vi "LDA_Analysis.vi"() -> (5 "Plug in titles":string[](array[string]), 7 "Plug in values":string[](array[string]))   [LabVIEW 2011]
uses:
  Controls/Save_Data.ctl
  Globals/LDA_meas_global_1.vi
  Globals/Plug_in_data_global.vi
  Globals/Meas_global.vi
  Globals/Constants_global.vi
  <vilib>/Analysis/NI_AALBase.lvlib
panel:
  in  "File Extension":string=".xls"
  out "Delta f":dbl
  in  "Refined Spectra":bool
  in  "No of estimates output":i32=300
  out "Autocorrelation":cluster{dbl, dbl, dbl[]}[](graph)
  in  "Mode":enum16{"Spectra", "Autocorrelation"}(ring)
  in  "Separation Character":string="\t"
  in  "Precision":i16=2
  out "Ch names":string[](array[string])
  out "Number or Good blocks":i32
  out "Resampled block length":i32
  out "Resampling Frequency":dbl
  in  "Output Directory":path
  in  "File":T1=enum."Save Data"
  out "Frequency Spectrum":cluster{dbl, dbl, dbl[]}[](graph)
  # "You must have just these two indicators on the connector pane of the vi"
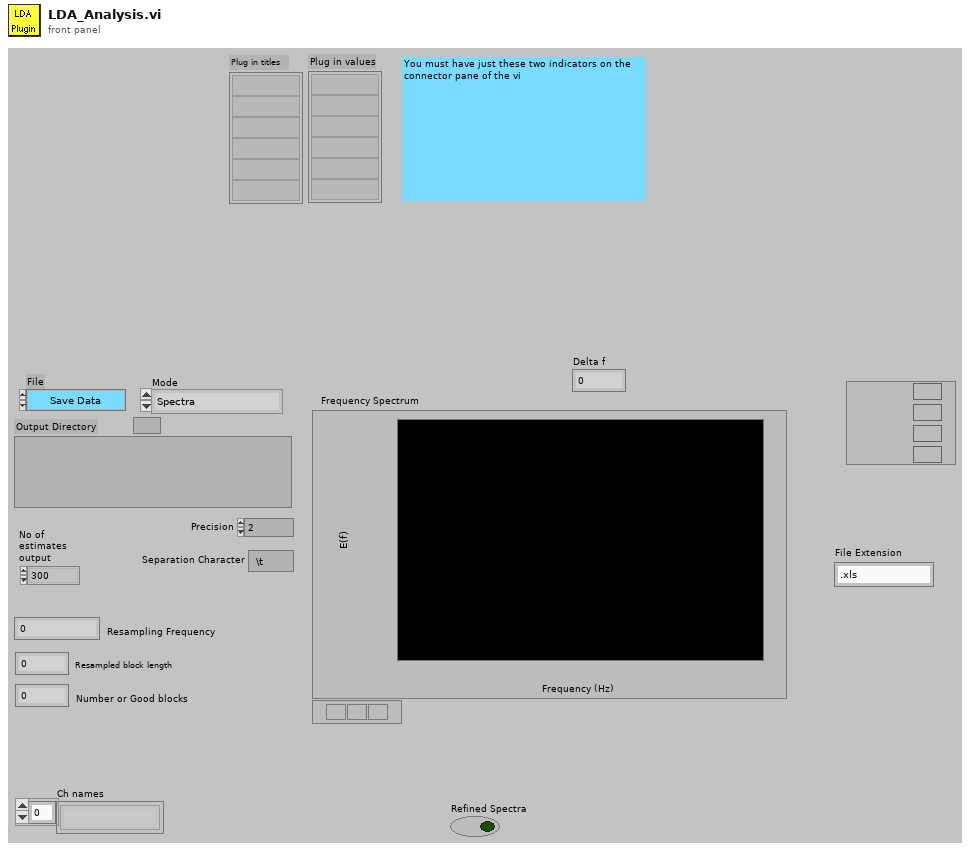
[diagram p1: front panel]
types:
  T1 = typedef "Save_Data.ctl" = enum16{"Save No Data", "Save Data"}
  T2 = enum32{"existing file", "new file", "new or existing file", "existing dir", "new dir", "new or existing dir", "existing file (use LLBs)", "new file (use LLBs)", "new or existing file (use LLBs)", "new or existing file or directory (use LLBs)"}
  T3 = typedef "Analysis_info_cluster.ctl" = cluster{"Colour":u32, "Inst type":T4, "Inst name":string, "Symbol":string, "Code name":string, "Extra Info":string, "Inst Array":T5, "Index":i32, "Voltage Index":i32, "Extra Titles":string[], "Extra Values":string[]}
  T4 = typedef "Inst_type.ctl" = enum16{"Propeller anemometer", "Raw voltage", "Pressure Transducer", "Pitot-static tube", "Preston tube", "Hot wire", "Cross wire 1", "Cross wire 2", "Generic Linear", "Generic Polynomial", "Generic BackPoly", "Fast FID", "Thermocouple", "Cold wire", "Pulsed Wire", "LDA Vel", "LDA Tran time", "LDA Arr time"}
  T5 = typedef "Instrument_Array.ctl" = enum16{"PWA", "LDA", "Analogue"}
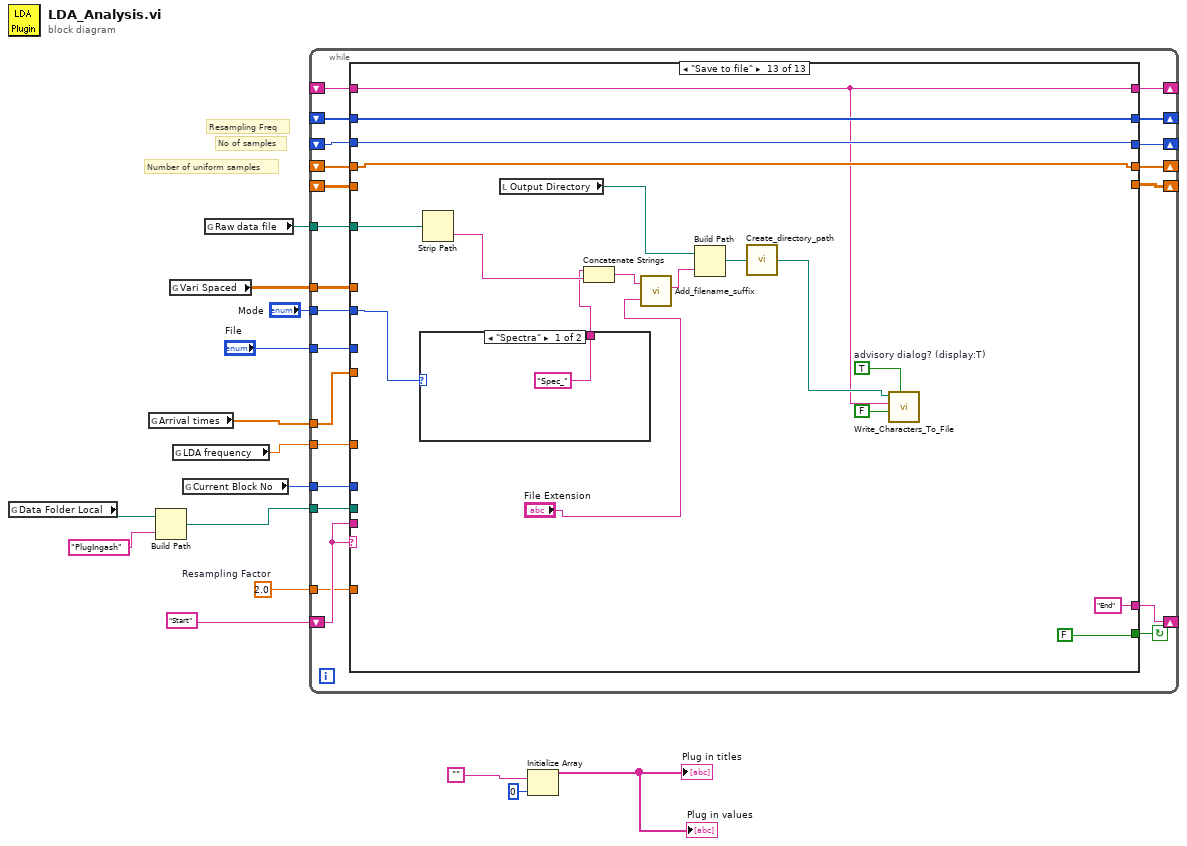
[diagram p0: block diagram]
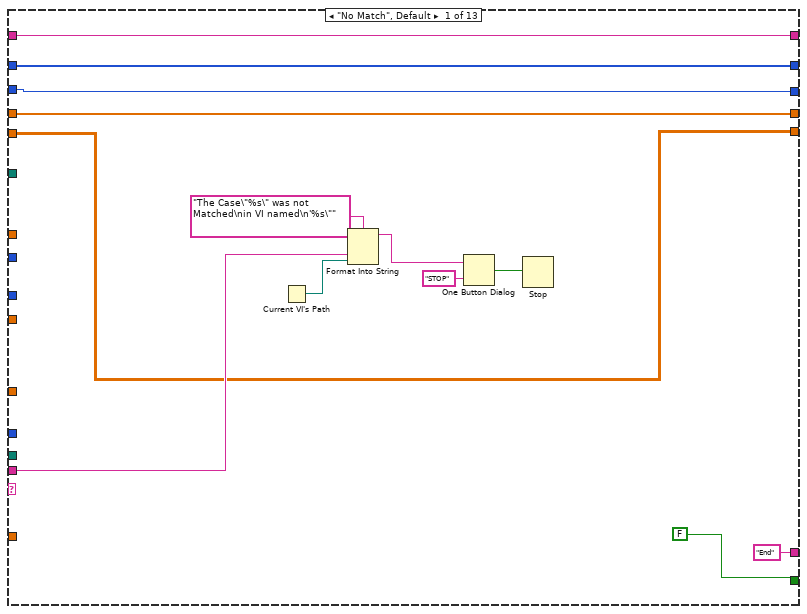
[diagram p2: hidden frame]
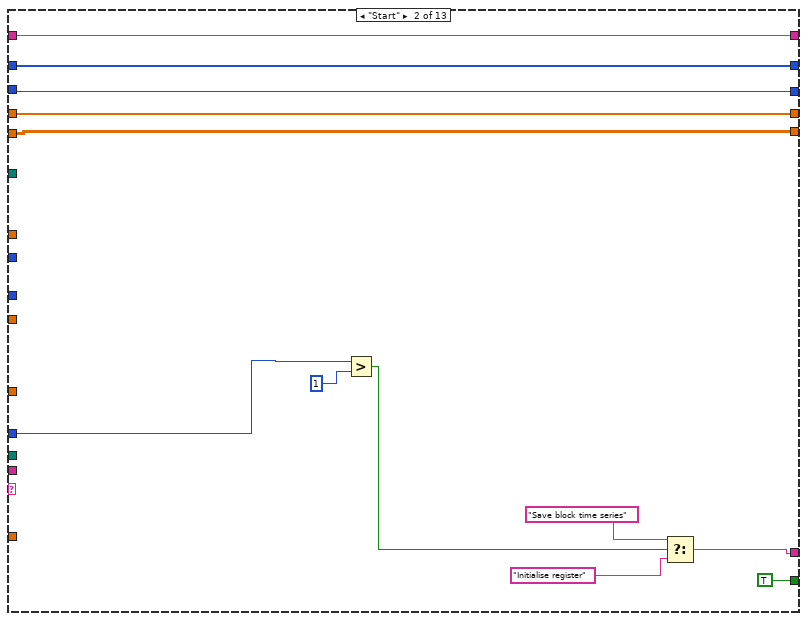
[diagram p3: hidden frame]
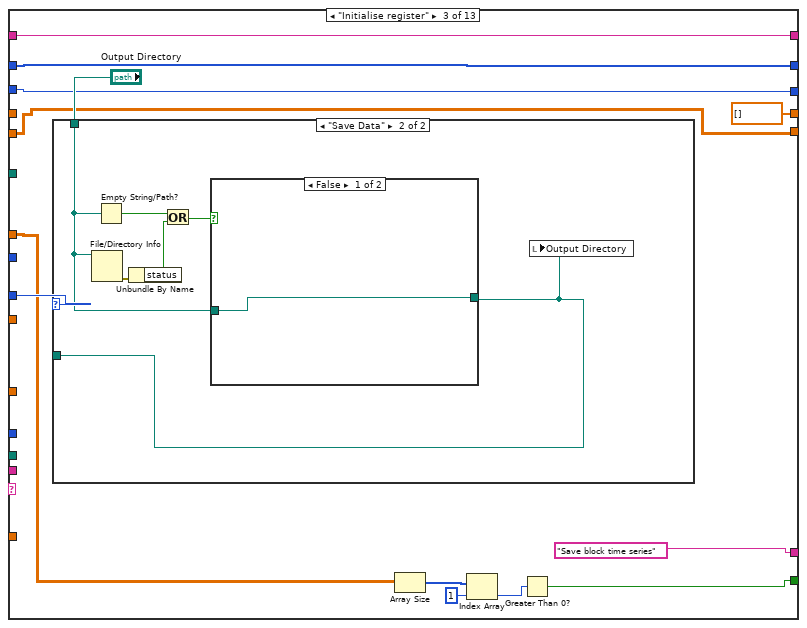
[diagram p4: hidden frame]
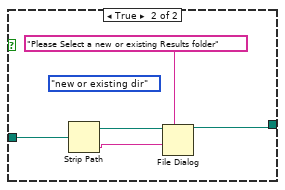
[diagram p6: hidden frame]
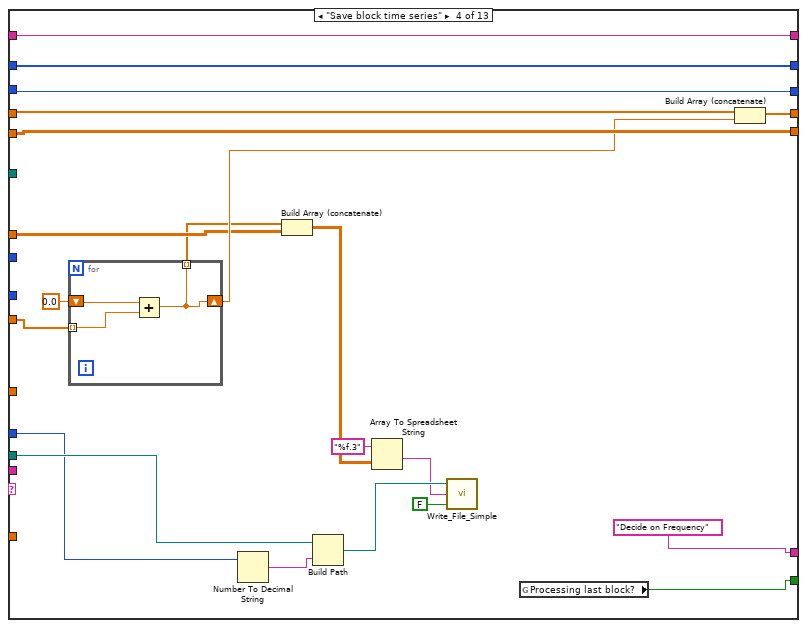
[diagram p7: hidden frame]
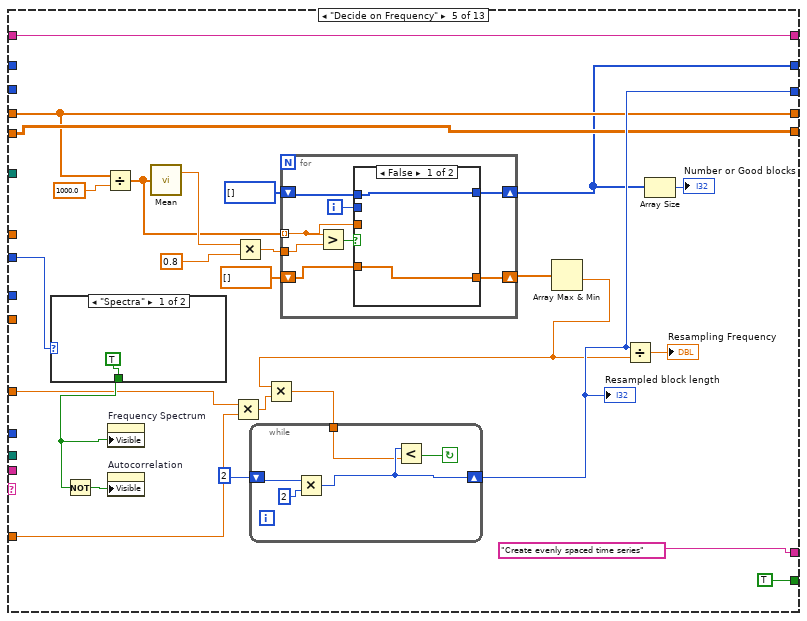
[diagram p8: hidden frame]
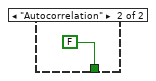
[diagram p9: hidden frame]
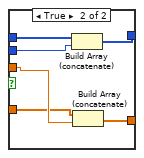
[diagram p10: hidden frame]
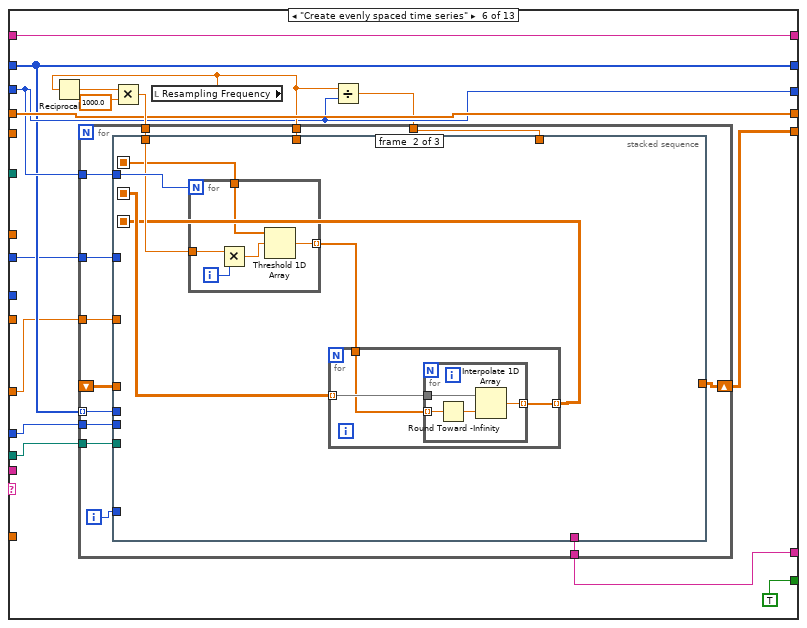
[diagram p11: hidden frame]
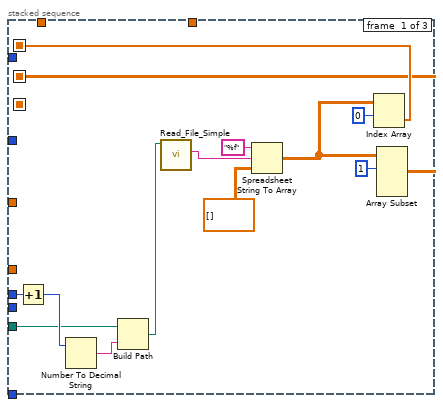
[diagram p12: hidden frame]
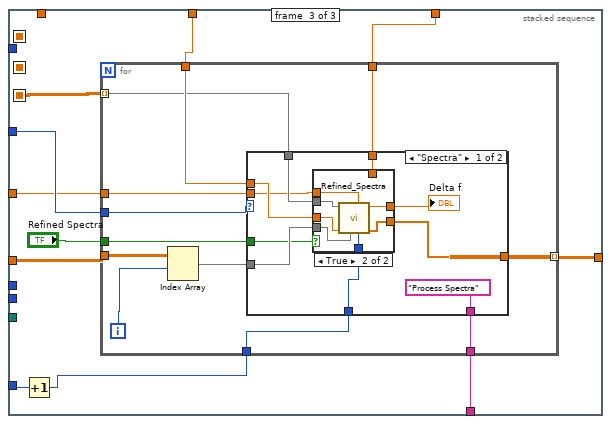
[diagram p13: hidden frame]
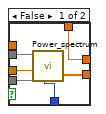
[diagram p14: hidden frame]
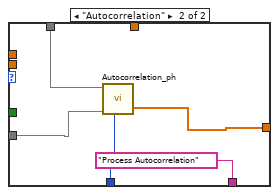
[diagram p15: hidden frame]
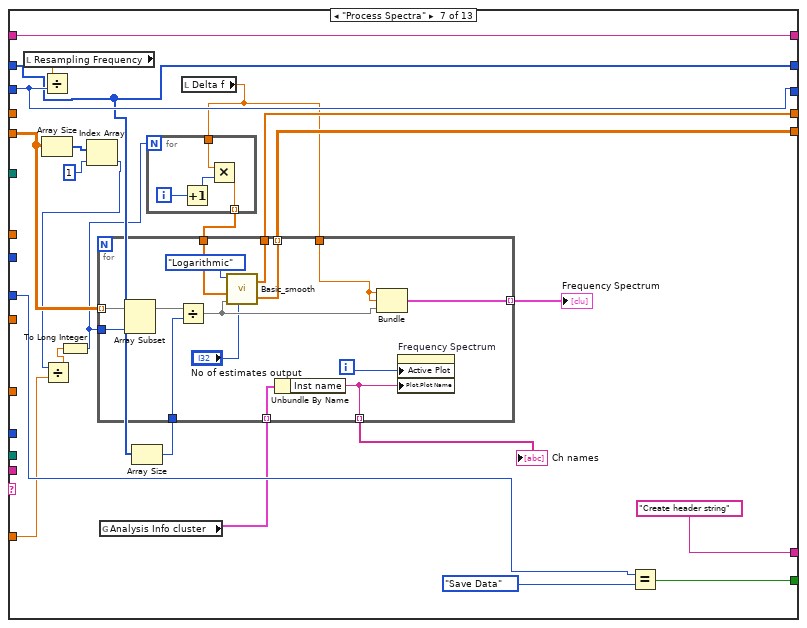
[diagram p16: hidden frame]
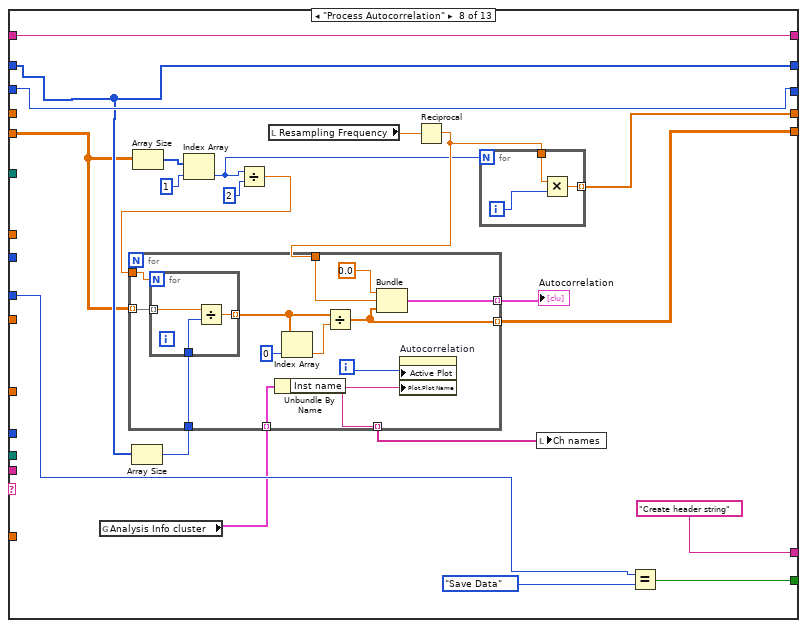
[diagram p17: hidden frame]
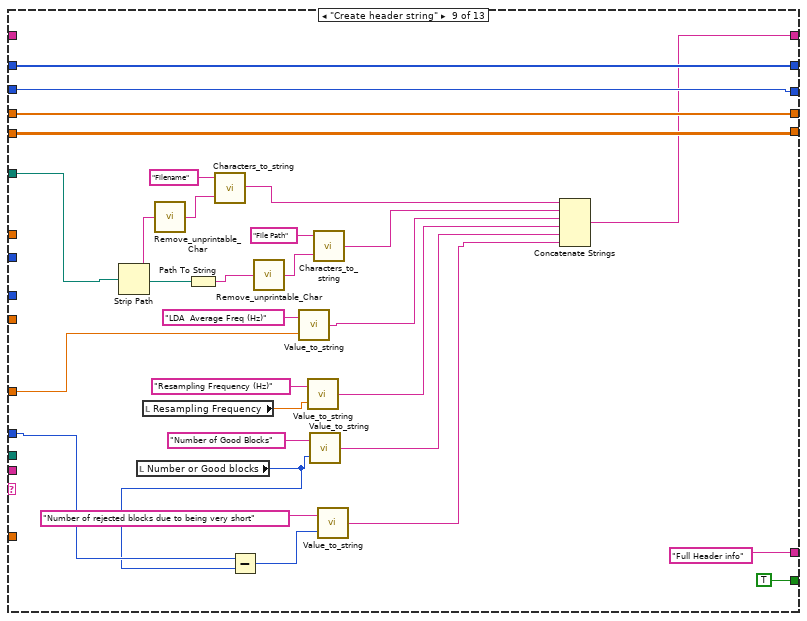
[diagram p18: hidden frame]
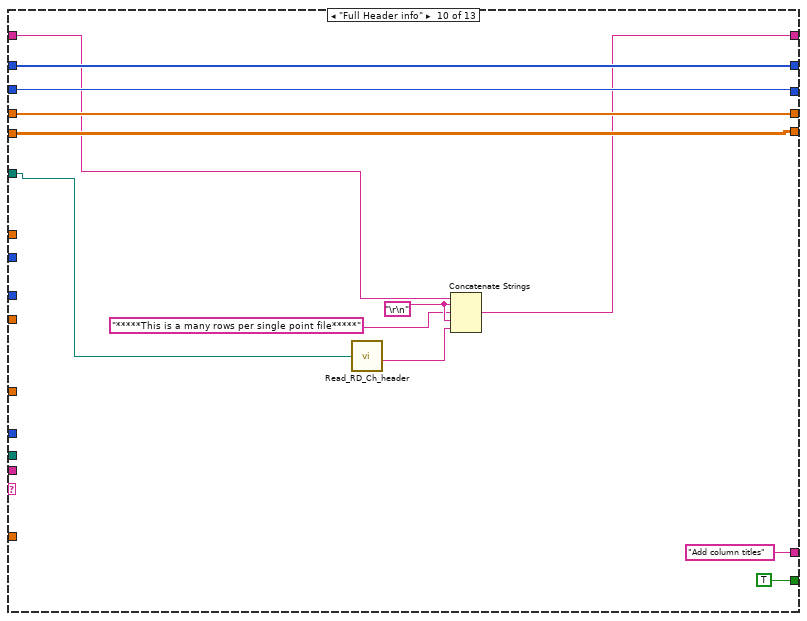
[diagram p19: hidden frame]
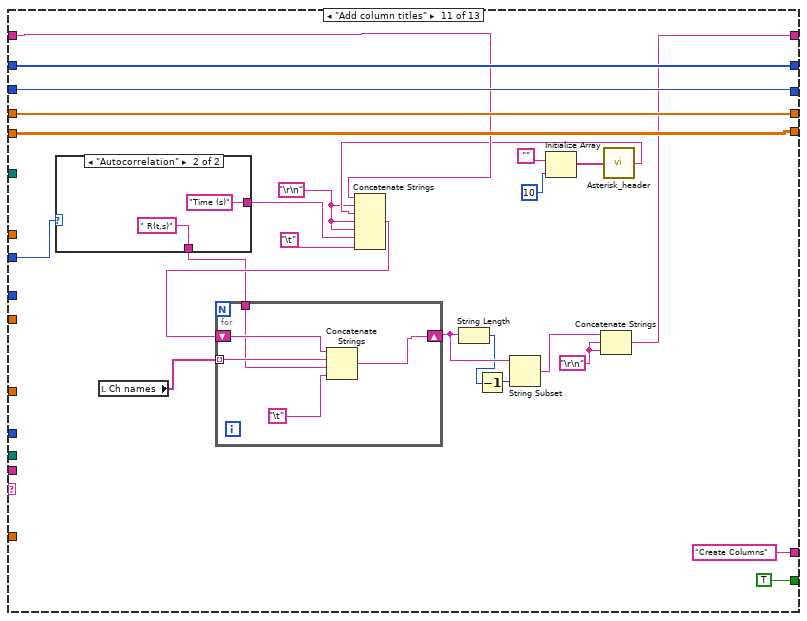
[diagram p20: hidden frame]
diagram:
  w1 = 2.0  # Resampling Factor
  # "No of samples"
  # "Number of uniform samples"
  # "Resampling Freq"
  n1 = global read "Constants_global.vi" "Data Folder Local"() -> (w7:path)
  n2 = global read "LDA_meas_global_1.vi" "Arrival times"() -> (w13:dbl[])
  n3 = Build Path(base path=w7, name or relative path="PlugIngash") -> (appended path=w6:path)
  n4 = global read "Plug_in_data_global.vi" "Vari Spaced"() -> (w14:dbl[][])
  n5 = global read "Meas_global.vi" "LDA frequency"() -> (w3:dbl)
  n6 = global read "Meas_global.vi" "Current Block No"() -> (w9:i32)
  n7 = global read "Meas_global.vi" "Raw data file"() -> (w4:path)
  n8 = while {
    shift-left: "Start" -> [w37]
    shift-right: [w34] -> _
    tunnel: w14 -> [w36]
    tunnel: w13 -> [w35]
    shift-right: [w32] -> _
    shift-left: _ -> [w31]
    shift-right: [w30] -> _
    shift-left: _ -> [w29]
    tunnel: w9 -> [w28]
    tunnel: w6 -> [w27]
    shift-right: [w26] -> _
    shift-left: _ -> [w25]
    tunnel: "File" -> [w24]
    shift-right: [w23] -> _
    shift-left: _ -> [w22]
    tunnel: w4 -> [w21]
    tunnel: w3 -> [w20]
    shift-right: [w19] -> _
    shift-left: _ -> [w18]
    tunnel: "Mode" -> [w17]
    tunnel: w1 -> [w16]
    stop <- w33 continue-if-true
    n9 = case shown="\"Save to file\"" w37 {
      tunnel: ["End" ("t") w57 "Save block time series" ("t") "Decide on Frequency" ("t") "Create evenly spaced time series" ("t") w164 "Create header string" "Create header string" "Full Header info" ("t") "Add column titles" ("t") "Create Columns" ("t") "Save to file" ("t") "End" ("t")] -> w34
      tunnel: w37 -> [w46 _ _ _ _ _ _ _ _ _ _ _ _]
      tunnel: w36 -> [_ _ w67 w90 _ _ _ _ _ _ _ _ _]
      tunnel: w35 -> [_ _ _ w96 _ _ _ _ _ _ _ _ _]
      tunnel: [FALSE TRUE w63 w101 TRUE TRUE ("Processing last block?") w290 w331 TRUE ("Processing last block?") TRUE ("Processing last block?") TRUE ("Processing last block?") TRUE ("Processing last block?") FALSE] -> w33
      tunnel: [w43 w53 w70 w97 w131 w173 w286 w325 w358 w393 w417 w435 _] -> w32
      tunnel: w31 -> [w43 w53 w70 w97 w131 _ w279 w322 w358 w393 w417 w435 _]
      tunnel: [w41 w56 dbl[] [] w99 w127 w172 w282 w316 w359 w394 w418 w430 w491] -> w30
      tunnel: w29 -> [w41 w56 _ w100 w127 w172 _ _ w359 w394 w418 w430 w491]
      tunnel: w28 -> [_ w55 _ w106 _ w162 _ _ w367 _ _ _ _]
      tunnel: w27 -> [_ _ _ w107 _ w175 _ _ _ _ _ _ _]
      tunnel: [w42 w54 w71 w98 w132 w169 w293 w334 w360 w395 w419 w437 w492] -> w26
      tunnel: w25 -> [w42 w54 w71 w98 _ w169 w293 w334 w360 w395 w419 w437 w492]
      tunnel: w24 -> [_ _ w72 _ _ _ w291 w332 _ _ _ _ _]
      tunnel: [w40 w52 w69 w93 w121 w167 w285 w328 w361 w396 w420 w445 w490] -> w23
      tunnel: w22 -> [w40 w52 w69 w93 _ w167 w285 w328 w361 w396 w420 w445 w490]
      tunnel: w21 -> [_ _ _ _ _ _ _ _ w373 w386 _ _ w489]
      tunnel: w20 -> [_ _ _ _ w114 w163 _ _ w370 _ _ _ _]
      tunnel: [w39 w51 w68 w92 w119 w166 w289 w330 w357 w385 w413 w441 w482] -> w19
      tunnel: w18 -> [w39 w51 w68 w92 w119 w166 w289 w330 _ w392 w407 w442 w482]
      tunnel: w17 -> [_ _ _ _ w118 w165 _ _ _ _ w410 _ w479]
      tunnel: w16 -> [_ _ _ _ w113 _ w275 _ _ _ _ _ _]
      frame "No Match", Default {
        n10 = Current VI's Path() -> (path=w45:path)
        n11 = Format Into String(format string="The Case\"%s\" was not Matched\nin VI named\n'%s\"" ("Format String"), w46, w45) -> (resulting string=w49:string)  [unwired: 2 in, 1 out]
        n12 = One Button Dialog(message=w49, button name ("OK")="STOP") -> (true=w47:bool)
        n13 = Stop(stop? (T)=w47) -> ()
      }
      frame "Start" {
        n14 = Greater?(x=w55, y=1) -> (0:w59:bool)
        n15 = Select(t="Save block time series", s=w59, f="Initialise register") -> (s? t:f=w57:string)
      }
      frame "Initialise register" {
        n16 = case shown="\"Save Data\"" w72 {
          tunnel: [w76 w82] -> _
          tunnel: "Output Directory" -> [w76 w80]
          frame "Save No Data" {
          }
          frame "Save Data" {
            n17 = File/Directory Info(path=w80) -> (error out=w81:errorcluster)  [unwired: 1 in, 6 out]
            n18 = Empty String/Path?(string/path=w80) -> (empty?=w78:bool)
            n19 = Unbundle By Name(w81) -> ("status"=w79:bool)
            n20 = Or(x=w78, y=w79) -> (x .or. y?=w77:bool)
            n21 = case shown="False" w77 {
              tunnel: [w83 w88] -> w82
              tunnel: w80 -> [w83 w86]
              frame False {
              }
              frame True {
                (unwired) T2."new or existing dir" ("select mode (2)")
                n22 = Strip Path(path=w86) -> (stripped path=w85:path, name=w84:string)
                n23 = File Dialog(7:"Please Select a new or existing Results folder" ("prompt"), 9:w84, 11:w85) -> (3:w88:path)  [unwired: 1 in, 6 out]
              }
            }
            n24 = local write "Output Directory"(w82) -> ()
          }
        }
        n25 = Array Size(array=w67) -> (size(s)=w66:i32[])
        n26 = Index Array(array=w66, index=1) -> (element=w64:i32)
        n27 = Greater Than 0?(x=w64) -> (x > 0?=w63:bool)
      }
      frame "Save block time series" {
        n28 = for {
          shift-right: [w110] -> w94
          shift-left: 0.0 -> [w112]
          tunnel: w96 -> [w111] mode=indexing
          tunnel: [w110] -> w89 mode=indexing
          n29 = Add(x=w112, y=w111) -> (x+y=w110:dbl)
        }
        n30 = Number To Decimal String(number=w106) -> (decimal integer string=w105:string)  [unwired: 1 out]
        n31 = Build Array (concatenate)(w89, w90) -> (w91:dbl[][])
        n32 = Build Path(base path=w107, name or relative path=w105) -> (appended path=w104:path)
        n33 = Array To Spreadsheet String(array=w91, 3:"%f.3" ("format string")) -> (spreadsheet string=w103:string)  [unwired: 1 out]
        n34 = call "Write_File_Simple.vi"("append to file? (new file:F)"=FALSE, "character string"=w103, "file path"=w104) -> ()  [unwired: 2 out]
        n35 = global read "Meas_global.vi" "Processing last block?"() -> (w101:bool)
        n36 = Build Array (concatenate)(w100, w94) -> (w99:dbl[])
      }
      frame "Decide on Frequency" {
        n37 = case shown="\"Spectra\"" w118 {
          tunnel: [TRUE FALSE] -> w116
          frame "Spectra" {
          }
          frame "Autocorrelation" {
          }
        }
        n38 = Not(x=w116) -> (.not. x?=w117:bool)
        n39 = Divide(x=w127, y=1000.0) -> (x/y=w125:dbl[])
        n40 = property on="Frequency Spectrum" class="WFGraph (strict)"("Visible"=w116) -> ()  [unwired: 2 in, 2 out]
        n41 = property on="Autocorrelation" class="WFGraph (strict)"("Visible"=w117) -> ()  [unwired: 2 in, 2 out]
        n42 = call <vilib>:"Mean.vi"("X"=w125) -> ("mean"=w130:dbl)  [unwired: 1 out]
        n43 = Multiply(x=w114, y=w113) -> (x*y=w115:dbl)
        n44 = Multiply(x=w130, y=0.8) -> (x*y=w128:dbl)
        n45 = for {
          tunnel: w125 -> [w143] mode=indexing
          tunnel: w128 -> [w148]
          shift-right: [w144] -> w121
          shift-left: i32[] [] -> [w145]
          shift-right: [w141] -> w123
          shift-left: dbl[] [] -> [w142]
          i -> [w146]
          n46 = Greater?(x=w143, y=w148) -> (0:w147:bool)
          n47 = case shown="False" w147 {
            tunnel: w146 -> [_ w156]
            tunnel: w145 -> [w150 w155]
            tunnel: [w150 w154] -> w144
            tunnel: w143 -> [_ w153]
            tunnel: w142 -> [w149 w152]
            tunnel: [w149 w151] -> w141
            frame False {
            }
            frame True {
              n48 = Build Array (concatenate)(w155, w156) -> (w154:i32[])
              n49 = Build Array (concatenate)(w152, w153) -> (w151:dbl[])
            }
          }
        }
        n50 = Array Max & Min(array=w123) -> (min value=w122:dbl)  [unwired: 3 out]
        n51 = Multiply(x=w122, y=w115) -> (x*y=w134:dbl)
        n52 = while {
          shift-right: [w159] -> w132
          shift-left: 2 -> [w161]
          tunnel: w134 -> [w158]
          stop <- w157 continue-if-true
          n53 = Multiply(x=w161, y=2) -> (x*y=w159:i32)
          n54 = Less?(x=w159, y=w158) -> (x < y?=w157:bool)
        }
        "Resampled block length" <- w132
        n55 = Divide(x=w132, y=w122) -> (x/y=→"Resampling Frequency":dbl)
        n56 = Array Size(array=w121) -> (size(s)=→"Number or Good blocks":i32)
      }
      frame "Create evenly spaced time series" {
        n57 = local read "Resampling Frequency"() -> (w170:dbl)
        n58 = Reciprocal(x=w170) -> (1/x=w176:dbl)
        n59 = Multiply(x=w176, y=1000.0) -> (x*y=w174:dbl)
        n60 = Divide(x=w170, y=w169) -> (x/y=w168:dbl)
        n61 = for {
          tunnel: w175 -> [w190]
          tunnel: w169 -> [w189]
          tunnel: w174 -> [w188]
          shift-right: [w186] -> w173
          shift-left: _ -> [w187]
          tunnel: w170 -> [w185]
          tunnel: w168 -> [w184]
          tunnel: w167 -> [w182] mode=indexing
          tunnel: w165 -> [w181]
          tunnel: [w180] -> w164
          tunnel: w163 -> [w179]
          tunnel: w162 -> [w178]
          i -> [w183]
          n62 = stacked-sequence {
            seq-local: [w196 _ _] -> [_ w207 _]
            seq-local: [w193 _ _] -> [_ w205 _]
            seq-local: [_ w204 _] -> [_ _ w232]
            tunnel: w183 -> [_ _ w228]
            tunnel: w190 -> [w201 _ _]
            tunnel: w189 -> [_ w209 _]
            tunnel: w188 -> [_ w208 _]
            tunnel: w187 -> [_ _ w231]
            tunnel: [_ _ w230] -> w186
            tunnel: w185 -> [_ _ w229]
            tunnel: w184 -> [_ _ w222]
            tunnel: w182 -> [w191 _ _]
            tunnel: w181 -> [_ _ w226]
            tunnel: [_ _ w225] -> w180
            tunnel: w179 -> [_ _ w224]
            tunnel: w178 -> [_ _ _]
            frame #0 {
              n63 = Increment(x=w191) -> (x+1=w202:i32)
              n64 = Number To Decimal String(number=w202) -> (decimal integer string=w203:string)  [unwired: 1 out]
              n65 = Build Path(base path=w201, name or relative path=w203) -> (appended path=w200:path)
              n66 = call "Read_File_Simple.vi"("Filename"=w200) -> ("string"=w199:string)  [unwired: 2 in, 7 out]
              n67 = Spreadsheet String To Array(format string="%f", spreadsheet string=w199, array type (2D Dbl)=dbl[][] []) -> (array=w195:dbl[][])  [unwired: 1 out]
              n68 = Index Array(array=w195, index (row)=0) -> (element=w196:dbl[])  [unwired: 1 in]
              n69 = Array Subset(array=w195, index (row)=1 ("index")) -> (w193:dbl[][])  [unwired: 3 in]
            }
            frame #1 {
              n70 = for {
                N: w209 -> [_]
                tunnel: w208 -> [w220]
                tunnel: w207 -> [w219]
                tunnel: [w218] -> w206 mode=indexing
                i -> [w221]
                n71 = Multiply(x=w220, y=w221) -> (x*y=w217:dbl)
                n72 = Threshold 1D Array(2:w217, 3:w219) -> (0:w218:dbl)  [unwired: 1 out]
              }
              n73 = for {
                tunnel: [w212] -> w204 mode=indexing
                tunnel: w206 -> [w210]
                tunnel: w205 -> [w211] mode=indexing
                n74 = for {
                  tunnel: w211 -> [w216]
                  tunnel: w210 -> [w215] mode=indexing
                  tunnel: [w214] -> w212 mode=indexing
                  n75 = Round Toward -Infinity(1:w215) -> (0:w213:dbl)
                  n76 = Interpolate 1D Array(1:w213, 2:w216) -> (0:w214:dbl)
                }
              }
            }
            frame #2 {
              n77 = Increment(x=w228) -> (x+1=w227:i32)
              n78 = for {
                tunnel: w232 -> [w240] mode=indexing
                tunnel: [w239] -> w230 mode=indexing
                tunnel: w231 -> [w244]
                tunnel: w229 -> [w241]
                tunnel: w227 -> [w238]
                tunnel: w226 -> [w237]
                tunnel: [w236] -> w225
                tunnel: w224 -> [w235]
                tunnel: "Refined Spectra" -> [w234]
                tunnel: w222 -> [w233]
                i -> [w242]
                n79 = Index Array(array=w244, index (row)=w242) -> (element=w243:dbl[])  [unwired: 1 in]
                n80 = case shown="\"Spectra\"" w237 {
                  tunnel: w243 -> [w254 w271]
                  tunnel: w241 -> [w249 _]
                  tunnel: w240 -> [w250 w272]
                  tunnel: [w253 w270] -> w239
                  tunnel: w238 -> [w252 w269]
                  tunnel: ["Process Spectra" ("t") "Process Autocorrelation" ("t")] -> w236
                  tunnel: w235 -> [w248 _]
                  tunnel: w234 -> [w247 _]
                  tunnel: w233 -> [w245 _]
                  frame "Spectra" {
                    n81 = case shown="True" w247 {
                      tunnel: w254 -> [w260 w264]
                      tunnel: [w259 w266] -> w253
                      tunnel: w252 -> [w258 w263]
                      tunnel: w250 -> [w257 w267]
                      tunnel: w249 -> [w256 w265]
                      tunnel: w248 -> [_ w262]
                      tunnel: [w255 w261] -> w246
                      tunnel: w245 -> [w255 _]
                      frame False {
                        n82 = call "Power_spectrum.vi"("U"=w257, "Sampling frequency"=w256, "Spectrum input array"=w260, "Block No"=w258) -> ("Spectrum output array"=w259:dbl[])  [unwired: 1 in, 1 out]
                      }
                      frame True {
                        n83 = call "Refined_Spectra.vi"("Block No"=w263, "LDA Frequency"=w262, "Spectrum input array"=w264, "Sampling frequency"=w265, "X"=w267) -> ("Spectrum"=w266:dbl[], "Delta f"=w261:dbl)  [unwired: 5 in]
                      }
                    }
                    "Delta f" <- w246
                  }
                  frame "Autocorrelation" {
                    n84 = call "Autocorrelation_ph.vi"("X"=w272, "Autocorrelation of X"=w271, "Block No"=w269) -> ("Autocorrelation of X"=w270:dbl[])  [unwired: 2 in, 1 out]
                  }
                }
              }
            }
          }
        }
      }
      frame "Process Spectra" {
        (unwired) FALSE
        n85 = local read "Resampling Frequency"() -> (w294:dbl)
        n86 = Divide(x=w294, y=w293) -> ()  [unwired: 1 out]
        n87 = Array Size(array=w279) -> (size(s)=w281:i32[])
        n88 = Index Array(array=w281, index=1) -> (element=w276:i32)
        n89 = Divide(x=w276, y=w275) -> (x/y=w274:dbl)
        n90 = To Long Integer(number=w274) -> (32bit integer=w273:i32)
        n91 = global read "Meas_global.vi" "Analysis Info cluster"() -> (w287:T3[])
        n92 = Array Size(array=w285) -> (size(s)=w284:i32)
        n93 = local read "Delta f"() -> (w278:dbl)
        n94 = for {
          N: w273 -> [_]
          tunnel: w278 -> [w297]
          tunnel: [w296] -> w283 mode=indexing
          i -> [w299]
          n95 = Increment(x=w299) -> (x+1=w298:i32)
          n96 = Multiply(x=w297, y=w298) -> (x*y=w296:dbl)
        }
        n97 = for {
          tunnel: w279 -> [w301] mode=indexing
          tunnel: w284 -> [w314]
          tunnel: [w313] -> w277 mode=indexing
          tunnel: w287 -> [w311] mode=indexing
          tunnel: [w310] -> w288 mode=indexing
          tunnel: [w305] -> w286 mode=indexing
          tunnel: w283 -> [w308]
          tunnel: [w304] -> w282
          tunnel: w278 -> [w303]
          tunnel: w273 -> [w300]
          i -> [w312]
          n98 = Array Subset(array=w301, length=w300) -> (w302:dbl[])  [unwired: 1 in]
          n99 = Divide(x=w302, y=w314) -> (x/y=w309:dbl[])
          n100 = call "Basic_smooth.vi"("Smoothing"=enum16{"Linear", "Logarithmic"}."Logarithmic", "X array in"=w308, "Y array in"=w309, "No of estimates output"="No of estimates output") -> ("X array Out"=w304:dbl[], "Y array Out"=w305:dbl[])  [unwired: 1 out]
          n101 = Unbundle By Name(w311) -> ("Inst name"=w310:string)
          n102 = Bundle("Delta f"=w303, "Delta f"=w303, w309) -> (w313:cluster{"Delta f":dbl, "Delta f":dbl, dbl[]})  [unwired: 1 out]
          n103 = property on="Frequency Spectrum" class="WFGraph (strict)"("Active Plot"=w312, "Plot.Plot Name"=w310) -> ()  [unwired: 2 in, 2 out]
        }
        "Frequency Spectrum" <- w277
        "Ch names" <- w288
        n104 = Equal?(x=w291, y=Save_Data."Save Data" ("File")) -> (x = y?=w290:bool)
      }
      frame "Process Autocorrelation" {
        (unwired) FALSE
        n105 = global read "Meas_global.vi" "Analysis Info cluster"() -> (w329:T3[])
        n106 = Array Size(array=w328) -> (size(s)=w327:i32)
        n107 = Array Size(array=w322) -> (size(s)=w321:i32[])
        n108 = Index Array(array=w321, index=1) -> (element=w315:i32)
        n109 = Divide(x=w315, y=2) -> (x/y=w318:dbl)
        n110 = local read "Resampling Frequency"() -> (w326:dbl)
        n111 = Reciprocal(x=w326) -> (1/x=w317:dbl)
        n112 = for {
          tunnel: w317 -> [w351]
          tunnel: w322 -> [w350] mode=indexing
          tunnel: w327 -> [w349]
          tunnel: [w348] -> w323 mode=indexing
          tunnel: w329 -> [w347] mode=indexing
          tunnel: [w342] -> w325 mode=indexing
          tunnel: [w340] -> w324 mode=indexing
          tunnel: w318 -> [w339]
          i -> [w341]
          n113 = for {
            N: w339 -> [_]
            tunnel: w350 -> [w354] mode=indexing
            tunnel: w349 -> [w353]
            tunnel: [w352] -> w344 mode=indexing
            n114 = Divide(x=w354, y=w353) -> (x/y=w352:dbl)
          }
          n115 = Unbundle By Name(w347) -> ("Inst name"=w340:string)
          n116 = Index Array(array=w344, index=0) -> (element=w343:dbl)
          n117 = Divide(x=w344, y=w343) -> (x/y=w342:dbl[])
          n118 = Bundle(0.0, w351, w342) -> (w348:cluster{dbl, dbl, dbl[]})  [unwired: 1 out]
          n119 = property on="Autocorrelation" class="WFGraph (strict)"("Active Plot"=w341, "Plot.Plot Name"=w340) -> ()  [unwired: 2 in, 2 out]
        }
        "Autocorrelation" <- w323
        n120 = for {
          N: w315 -> [_]
          tunnel: w317 -> [w338]
          tunnel: [w336] -> w316 mode=indexing
          i -> [w337]
          n121 = Multiply(x=w338, y=w337) -> (x*y=w336:dbl)
        }
        n122 = local write "Ch names"(w324) -> ()
        n123 = Equal?(x=w332, y=Save_Data."Save Data" ("File")) -> (x = y?=w331:bool)
      }
      frame "Create header string" {
        n124 = Strip Path(path=w373) -> (stripped path=w377:path, name=w381:string)
        n125 = local read "Number or Good blocks"() -> (w366:i32)
        n126 = local read "Resampling Frequency"() -> (w369:dbl)
        n127 = call "Remove_unprintable_Char.vi"("Input String"=w381) -> ("Output String"=w380:string)
        n128 = Path To String(path=w377) -> (string=w376:string)
        n129 = call "Characters_to_string.vi"("Characters to write"=w380, "Label for characters"="Filename") -> ("Output string"=w375:string)
        n130 = Subtract(x=w367, y=w366) -> (x-y=w365:i32)
        n131 = call "Remove_unprintable_Char.vi"("Input String"=w376) -> ("Output String"=w379:string)
        n132 = call "Value_to_string.vi"("Value"=w370, "Label for value"="LDA  Average Freq (Hz)") -> ("Output string"=w384:string)  [unwired: 1 in]
        n133 = call "Value_to_string.vi"("Value"=w369, "Label for value"="Resampling Frequency (Hz)") -> ("Output string"=w364:string)  [unwired: 1 in]
        n134 = call "Value_to_string.vi"("Value"=w366, "Label for value"="Number of Good Blocks") -> ("Output string"=w363:string)  [unwired: 1 in]
        n135 = call "Characters_to_string.vi"("Characters to write"=w379, "Label for characters"="File Path") -> ("Output string"=w374:string)
        n136 = call "Value_to_string.vi"("Value"=w365, "Label for value"="Number of rejected blocks due to being very short") -> ("Output string"=w362:string)  [unwired: 1 in]
        n137 = Concatenate Strings(w375, w374, w384, w364, w363, w362) -> (w357:string)
      }
      frame "Full Header info" {
        w389 = "\r\n"
        n138 = call "Read_RD_Ch_header.vi"("Raw data file"=w386) -> ("Ch string"=w387:string)  [unwired: 3 out]
        n139 = Concatenate Strings(w392, w389, "*****This is a many rows per single point file*****", w389, w387) -> (w385:string)
      }
      frame "Add column titles" {
        w401 = "\r\n"
        w402 = "\r\n"
        n140 = case shown="\"Autocorrelation\"" w410 {
          tunnel: ["f (Hz)" "Time (s)"] -> w409
          tunnel: [" E(f)" " R(t,s)"] -> w408
          frame "Spectra" {
          }
          frame "Autocorrelation" {
          }
        }
        n141 = local read "Ch names"() -> (w415:string[])
        n142 = Initialize Array("", 10) -> (w406:string[])
        n143 = call "Asterisk_header.vi"("Channel names"=w406) -> ("Header string"=w403:string)
        n144 = Concatenate Strings(w407, w401, w403, w401, w401, w409, "\t") -> (w414:string)
        n145 = for {
          shift-right: [w426] -> w400
          shift-left: w414 -> [w428]
          tunnel: w415 -> [w429] mode=indexing
          tunnel: w408 -> [w425]
          n146 = Concatenate Strings(w428, w429, w425, "\t") -> (w426:string)
        }
        n147 = String Length(string=w400) -> (length=w397:i32)
        n148 = Decrement(x=w397) -> (x-1=w398:i32)
        n149 = String Subset(string=w400, length (rest)=w398) -> (substring=w399:string)  [unwired: 1 out]
        n150 = Concatenate Strings(w399, w402, w402) -> (w413:string)
      }
      frame "Create Columns" {
        n151 = Array Size(array=w435) -> (size(s)=w433:i32[])
        n152 = Index Array(array=w433, index=0) -> (element=w432:i32)
        n153 = Decrement(x=w432) -> (x-1=w431:i32)
        n154 = for {
          shift-right: [w459] -> w440
          shift-left: "" -> [w454]
          tunnel: "Separation Character" -> [w447]
          tunnel: w435 -> [w457]
          tunnel: w431 -> [w453]
          tunnel: "Precision" -> [w451]
          tunnel: "Precision" -> [w450]
          tunnel: w430 -> [w446] mode=indexing
          i -> [w452]
          n155 = Index Array(array=w457, index (col)=w452) -> (element=w456:dbl[])  [unwired: 1 in]
          n156 = Number To Fractional String(number=w446, precision (6)=w450) -> (F-format string=w449:string)  [unwired: 2 out]
          n157 = Concatenate Strings(w449, w447) -> (w448:string)
          n158 = for {
            shift-right: [w466] -> w455
            shift-left: w448 -> [w468]
            tunnel: w447 -> [w465]
            tunnel: w456 -> [w460] mode=indexing
            tunnel: w453 -> [w463]
            tunnel: w451 -> [w461]
            i -> [w464]
            n159 = Equal?(x=w464, y=w463) -> (x = y?=w462:bool)
            n160 = Number To Exponential String(number=w460, precision (6)=w461) -> (E-format string=w467:string)  [unwired: 2 out]
            n161 = case shown="True" w462 {
              tunnel: w468 -> [w472 w475]
              tunnel: w467 -> [w471 w474]
              tunnel: [w470 w473] -> w466
              tunnel: w465 -> [w469 _]
              frame False {
                n162 = Concatenate Strings(w472, w471, w469) -> (w470:string)
              }
              frame True {
                n163 = Concatenate Strings(w475, w474) -> (w473:string)
              }
            }
          }
          n164 = Concatenate Strings(w454, w455, "\r\n") -> (w459:string)
        }
        n165 = Concatenate Strings(w442, w440) -> (w441:string)
      }
      frame "Save to file" {
        w484 = TRUE  # advisory dialog? (display:T)
        n166 = case shown="\"Spectra\"" w479 {
          tunnel: ["Spec_" ("string") "Auto_" ("string")] -> w480
          frame "Spectra" {
          }
          frame "Autocorrelation" {
          }
        }
        n167 = Strip Path(path=w489) -> (name=w487:string)  [unwired: 1 out]
        n168 = local read "Output Directory"() -> (w488:path)
        n169 = Concatenate Strings(w480, w487) -> (w478:string)
        n170 = call "Add_filename_suffix.vi"("Filename"=w478, "Suffix to add"="File Extension") -> ("Filename out"=w476:string)  [unwired: 3 out]
        n171 = Build Path(base path=w488, name or relative path=w476) -> (appended path=w486:path)
        n172 = call "Create_directory_path.vi"("Path name"=w486) -> ("Path name Out"=w485:path)
        n173 = call "Write_Characters_To_File.vi"("file path (dialog if empty)"=w485, "advisory dialog? (display:T)"=w484, "character string"=w482, "append to file? (new file:F)"=FALSE) -> ()  [unwired: 1 in, 4 out]
      }
    }
  }
  n174 = Initialize Array("", 0) -> (→"Plug in values" →"Plug in titles":string[])
